vi "niDTS BT Dut Rx Configure.vi"(0 "Dut Handle in":T2, 5 "niDTS BT DUT Parameters":T1={"Channel"=3, "Pattern"=enum."PN9", "Packet type"=enum."DH1", "Power"=0.0, "Report Period (ms)"=1000.0, "BD Address"=0, "Data Rate"=enum."1", "Number of Packets"=1500, "Packet Length, bytes"=1500} {"BD Address" format="%x"}, 7 "Apply Additional Defaults":bool=TRUE, 11 "error in (no error)":errorcluster) -> (4 "Dut Handle":T2, 15 "error out":errorcluster)   [LabVIEW 2015, in "niDTS BT.lvlib"]
doc: "Set the basic parameters for the WLAN TX Test. \n\nInputs:\n* Apply Additional Defaults. This allows more advanced parameters, which are dependant on the inputs, to have their default values set.\n\nCallbacks:\n* WLAN DUT Additional Defaults\n\nNote: This behavior is expected to be depricated when full parameter sets are passed as inputs and the input dependant defaults are calculated on the top parameter setting level."
uses:
  niDTS BT.lvlib
  Framework/Dut/Includes/niDTS Dut INC Handle.ctl
  Framework/Dut/Objects/BASE_class/niDTS Dut.lvclass
  Includes/niDTS BT DUT INC Parameters.ctl
  Includes/niDTS BT Dut INC Handle.ctl
  Objects/BASE_class/niDTS BT Dut.lvclass
  Includes/niDTS BT INC Standard.ctl
  Framework/Logger/Objects/BASE_class/niDTS Logger.lvclass
  Framework/niDTS Framework.lvlib
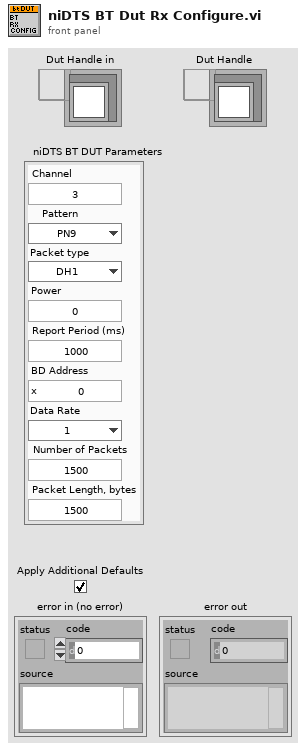
[diagram p1: front panel]
types:
  T1 = typedef "niDTS BT.lvlib/niDTS BT DUT INC Parameters.ctl" = cluster{"Channel":i32, "Pattern":enum16{"0", "1", "01", "00001111", "PN9"}, "Packet type":enum16{"NULL", "POLL", "FHS", "DM1", "DH1", "HV1", "HV2", "HV3", "EV3", "DV", "AUX1", "DM3", "DH3", "EV4", "EV5", "DM5", "DH5", "LE-TP"}, "Power":dbl, "Report Period (ms)":dbl, "BD Address":i64, "Data Rate":enum16{"1", "2", "3"}, "Number of Packets":i32, "Packet Length, bytes":i32}
  T2 = typedef "niDTS Framework.lvlib/niDTS Dut INC Handle.ctl" = refnum<data-value>
  T3 = typedef "niDTS BT.lvlib/niDTS BT INC Standard.ctl" = enum16{"BDR", "EDR", "LE-TP"}
  T4 = typedef "niDTS BT.lvlib/niDTS BT Dut INC Handle.ctl" = refnum<data-value>
  T5 = enum16{"NULL", "POLL", "FHS", "DM1", "DH1", "HV1", "HV2", "HV3", "EV3", "DV", "AUX1", "DM3", "DH3", "EV4", "EV5", "DM5", "DH5", "LE-TP"}
  T6 = typedef "niDTS Framework.lvlib/niDTS Logger INC Handle.ctl" = refnum<data-value>
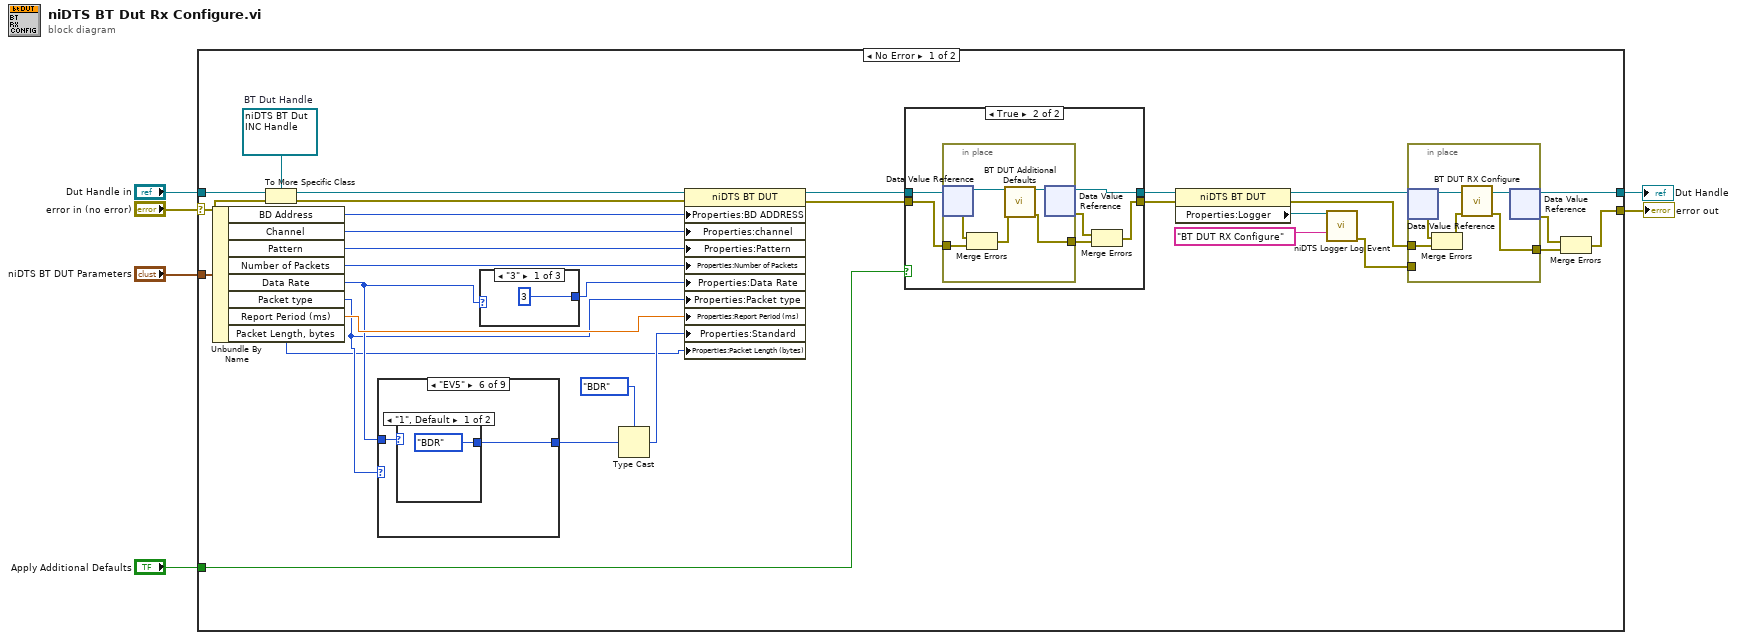
[diagram p0: block diagram]
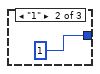
[diagram p2: hidden frame]
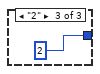
[diagram p3: hidden frame]
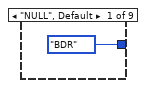
[diagram p4: hidden frame]
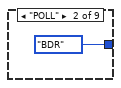
[diagram p5: hidden frame]
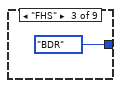
[diagram p6: hidden frame]
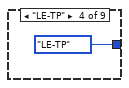
[diagram p7: hidden frame]
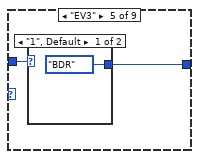
[diagram p8: hidden frame]
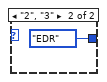
[diagram p9: hidden frame]
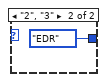
[diagram p10: hidden frame]
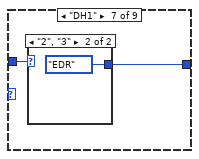
[diagram p11: hidden frame]
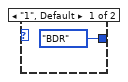
[diagram p12: hidden frame]
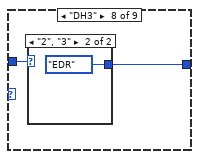
[diagram p13: hidden frame]
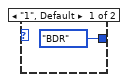
[diagram p14: hidden frame]
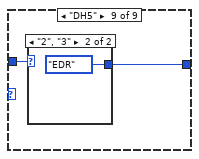
[diagram p15: hidden frame]
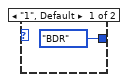
[diagram p16: hidden frame]
diagram:
  n1 = case shown="No Error" "error in (no error)" {
    selector: "error in (no error)" -> [w31 w86]
    tunnel: "Dut Handle in" -> [w38 w87]
    tunnel: "niDTS BT DUT Parameters" -> [w35 _]
    tunnel: "Apply Additional Defaults" -> [w34 _]
    tunnel: [w30 w87] -> w3
    tunnel: [w27 w86] -> w2
    frame No Error {
      w19 = T4 refnum  # BT Dut Handle
      n2 = Unbundle By Name(w35) -> ("BD Address"=w18:i64, "Channel"=w17:i32, "Pattern"=w16:enum16{"0", "1", "01", "00001111", "PN9"}, "Number of Packets"=w15:i32, "Data Rate"=w10:enum16{"1", "2", "3"}, "Packet type"=w8:T5, "Report Period (ms)"=w14:dbl, "Packet Length, bytes"=w7:i32)
      n3 = To More Specific Class(target class=w19, reference=w38, error in=w31) -> (specific class reference=w37:T4, error out=w36:errorcluster)
      n4 = case shown="\"EV5\"" w8 {
        tunnel: w10 -> [_ _ _ _ w47 w51 w55 w59 w63]
        tunnel: [niDTS_BT_INC_Standard."BDR" ("BT Standard") niDTS_BT_INC_Standard."BDR" ("BT Standard") niDTS_BT_INC_Standard."BDR" ("BT Standard") niDTS_BT_INC_Standard."LE-TP" ("BT Standard") w46 w50 w54 w58 w62] -> w12
        frame "NULL", Default {
        }
        frame "POLL" {
        }
        frame "FHS" {
        }
        frame "LE-TP" {
        }
        frame "EV3" {
          n5 = case shown="\"1\", Default" w47 {
            tunnel: [niDTS_BT_INC_Standard."BDR" ("BT Standard") niDTS_BT_INC_Standard."EDR" ("BT Standard")] -> w46
            frame "1", Default {
            }
            frame "2", "3" {
            }
          }
        }
        frame "EV5" {
          n6 = case shown="\"1\", Default" w51 {
            tunnel: [niDTS_BT_INC_Standard."BDR" ("BT Standard") niDTS_BT_INC_Standard."EDR" ("BT Standard")] -> w50
            frame "1", Default {
            }
            frame "2", "3" {
            }
          }
        }
        frame "DH1" {
          n7 = case shown="\"2\", \"3\"" w55 {
            tunnel: [niDTS_BT_INC_Standard."BDR" ("BT Standard") niDTS_BT_INC_Standard."EDR" ("BT Standard")] -> w54
            frame "1", Default {
            }
            frame "2", "3" {
            }
          }
        }
        frame "DH3" {
          n8 = case shown="\"2\", \"3\"" w59 {
            tunnel: [niDTS_BT_INC_Standard."BDR" ("BT Standard") niDTS_BT_INC_Standard."EDR" ("BT Standard")] -> w58
            frame "1", Default {
            }
            frame "2", "3" {
            }
          }
        }
        frame "DH5" {
          n9 = case shown="\"2\", \"3\"" w63 {
            tunnel: [niDTS_BT_INC_Standard."BDR" ("BT Standard") niDTS_BT_INC_Standard."EDR" ("BT Standard")] -> w62
            frame "1", Default {
            }
            frame "2", "3" {
            }
          }
        }
      }
      n10 = case shown="\"3\"" w10 {
        tunnel: [3 ("Data Rate") 1 ("Data Rate") 2 ("Data Rate")] -> w9
        frame "3" {
        }
        frame "1" {
        }
        frame "2" {
        }
      }
      n11 = Type Cast(type=enum16{"BDR", "EDR", "LE"}."BDR" ("Standard"), x=w12) -> (*(type *) &x=w11:enum16{"BDR", "EDR", "LE"})
      n12 = property class="niDTS BT DUT"(reference=w37, error in=w36, "Properties:BD ADDRESS"=w18, "Properties:channel"=w17, "Properties:Pattern"=w16, "Properties:Number of Packets"=w15, "Properties:Data Rate"=w9, "Properties:Packet type"=w8, "Properties:Report Period (ms)"=w14, "Properties:Standard"=w11, "Properties:Packet Length (bytes)"=w7) -> (reference out=w33:T4, error out=w32:errorcluster)
      n13 = case shown="True" w34 {
        tunnel: w33 -> [w73 w79]
        tunnel: w32 -> [w72 w78]
        tunnel: [w73 w75] -> w26
        tunnel: [w72 w74] -> w25
        frame False {
        }
        frame True {
          n14 = in-place {
            in-place-border: [w83] -> w77
            in-place-border: w78 -> [w82]
            n15 = in-place-dvr #1(w79) -> (w85:refnum<class "niDTS BT Dut.lvclass">, w81:errorcluster)
            n16 = Merge Errors(w81, w82) -> (w80:errorcluster)
            n17 = call-dynamic "BT DUT Additional Defaults.vi"("niDTS BT DUT in"=w85, "error in (no error)"=w80) -> ("niDTS BT DUT out"=w84:refnum<class "niDTS BT Dut.lvclass">, "error out"=w83:errorcluster)  [unwired: 12 in]
            n18 = in-place-dvr #1(w84) -> (w75:T4, w76:errorcluster)
          }
          n19 = Merge Errors(w76, w77) -> (w74:errorcluster)
        }
      }
      n20 = property class="niDTS BT DUT"(reference=w26, error in=w25) -> (reference out=w22:T4, error out=w21:errorcluster, "Properties:Logger"=w24:T6)
      n21 = call "niDTS Logger Log Event.vi"("Logger Handle"=w24, "Source/Location"="BT DUT RX Configure") -> ("error out"=w20:errorcluster)  [unwired: 11 in, 2 out]
      n22 = in-place {
        in-place-border: w21 -> [w71]
        in-place-border: [w66] -> w29
        in-place-border: w20 -> [_]
        n23 = in-place-dvr #2(w22) -> (w69:refnum<class "niDTS BT Dut.lvclass">, w70:errorcluster)
        n24 = Merge Errors(w70, w71) -> (w68:errorcluster)
        n25 = call-dynamic "BT DUT RX Configure.vi"("niDTS BT DUT in"=w69, "error in (no error)"=w68) -> ("niDTS BT DUT out"=w67:refnum<class "niDTS BT Dut.lvclass">, "error out"=w66:errorcluster)  [unwired: 12 in]
        n26 = in-place-dvr #2(w67) -> (w30:T4, w28:errorcluster)
      }
      n27 = Merge Errors(w28, w29) -> (w27:errorcluster)
    }
    frame Error {
    }
  }
  "error out" <- w2
  "Dut Handle" <- w3
